vi "Configure Date Basic.vi"(0 "VISA resource name":refnum<visa-resource-name>, 5 "Time Deviation Limit (5s)":u16(ring)=1 items=["Off", "5s", "10s", "15s"], 7 "Enable Change (Disable)":bool, 11 "error in (no error)":errorcluster) -> (4 "VISA resource name out":refnum<visa-resource-name>, 15 "error out":errorcluster)   [LabVIEW 2020, in "Yokogawa GX Series.lvlib"]
doc: "Sets the gradual time adjustment feature.\n\nCommand: SDateBasic"
uses:
  <instrlib>/Yokogawa GX Series/Yokogawa GX Series.lvlib
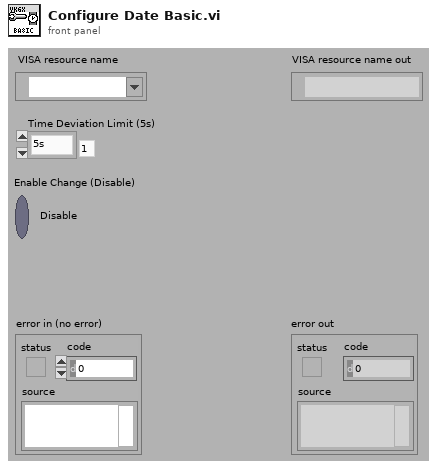
[diagram p1: front panel]
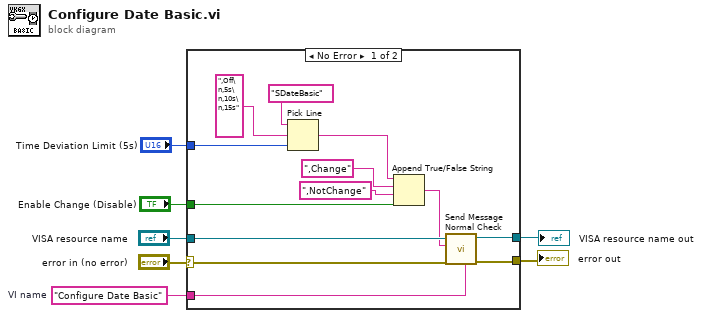
[diagram p0: block diagram]
diagram:
  w6 = "Configure Date Basic"  # VI name
  n1 = case shown="No Error" "error in (no error)" {
    selector: "error in (no error)" -> [w8 w21]
    tunnel: "VISA resource name" -> [w20 w22]
    tunnel: w6 -> [w19 _]
    tunnel: [w18 w22] -> w5
    tunnel: [w17 w21] -> w4
    tunnel: "Time Deviation Limit (5s)" -> [w16 _]
    tunnel: "Enable Change (Disable)" -> [w12 _]
    frame No Error {
      n2 = Pick Line(string ("")="SDateBasic", multi-line string=",Off\n,5s\n,10s\n,15s", line index=w16) -> (output string=w13:string)
      n3 = Append True/False String(1:w12, 2:",NotChange", 3:",Change", 4:w13) -> (0:w9:string)
      n4 = call <instrlib>:"Send Message Normal Check.vi"("Source (\"\")"=w19, "error in (no error)"=w8, "Send Message (\"\")"=w9, "VISA resource name"=w20) -> ("error out"=w17:errorcluster, "VISA resource name out"=w18:refnum<visa-resource-name>)  [unwired: 2 in, 4 out]
    }
    frame Error {
    }
  }
  "error out" <- w4
  "VISA resource name out" <- w5
